vi "Slider Get Offset.vi"(9 "Index":i32, 10 "LBCB Number":T1, 11 "DofType":T2) -> (2 "Offset":dbl)   [LabVIEW 2009]
uses:
  Data Access Objects/Limits/DofTypes.ctl
  Data Access Objects/Metadata/LBCB Number.ctl
  Global Data/Cartesian Measurment Actions.ctl
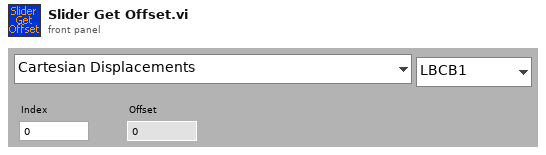
[diagram p1: front panel]
types:
  T1 = typedef "LBCB Number.ctl" = enum16{"LBCB1", "LBCB2"}
  T2 = typedef "DofTypes.ctl" = enum16{"Cartesian Displacements", "Cartesian Forces & Moments", "Actuator Displacements", "Actuator Forces"}
  T3 = typedef "Cartesian Measurment Actions.ctl" = enum16{"Set Data", "Get", "Init", "Set Offsets"}
  T4 = typedef "Cartesian Data Type.ctl" = cluster{"Displacements":dbl[], "Forces":dbl[], "Displacement Commands":dbl[]}
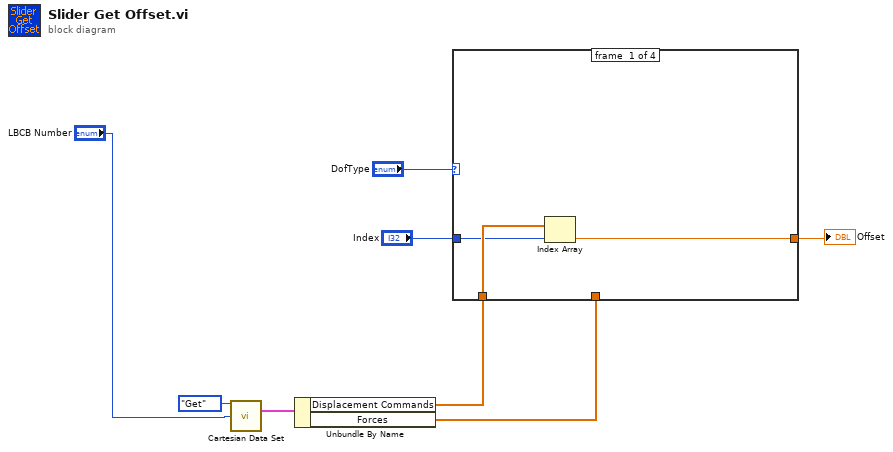
[diagram p0: block diagram]
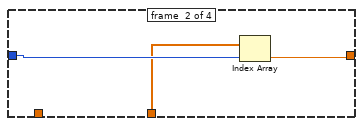
[diagram p2: hidden frame]
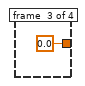
[diagram p3: hidden frame]
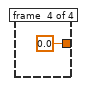
[diagram p4: hidden frame]
diagram:
  n1 = call "Cartesian Data Set.vi"("Measurement Actions"=Cartesian_Measurment_Actions."Get", "LBCB Selected"="LBCB Number") -> ("Cartesian Data Offsets Out"=w7:T4)  [unwired: 10 in, 3 out]
  n2 = Unbundle By Name(w7) -> ("Displacement Commands"=w4:dbl[], "Forces"=w3:dbl[])
  n3 = case shown="\"Actuator Displacements\"" "DofType" {
    tunnel: w4 -> [w11 _ _ _]
    tunnel: w3 -> [_ w12 _ _]
    tunnel: "Index" -> [w10 w14 _ _]
    tunnel: [w9 w13 0.0 ("Numeric") 0.0 ("Numeric")] -> w1
    frame #0 {
      n4 = Index Array(array=w11, index=w10) -> (element=w9:dbl)
    }
    frame #1 {
      n5 = Index Array(array=w12, index=w14) -> (element=w13:dbl)
    }
    frame #2 {
    }
    frame #3 {
    }
  }
  "Offset" <- w1
